vi "Lookup Class by ID (String).vi"(8 "error in (no error)":errorcluster, 11 "Class ID":string) -> (0 "error out":errorcluster, 2 "Found?":bool, 3 "Class Information":T1)   [LabVIEW 2023]
doc: "<b> </b> <b> </b>\n© 2017 Q Software Innovations, LLC\nwritten by Quentin \"Q\" Alldredge\nproduced in LabVIEW 2015\n\nsupport@qsoftwareinnovations.com\nwww.qsoftwareinnovations.com\n\nAll rights reserved.\n\nRedistribution and use in source and binary forms, with or without modification, are permitted provided that the following conditions are met:\n\n * Redistributions of source code must retain the above copyright notice, this list of conditions and the following disclaimer.\n * Redistributions in binary form must reproduce the above copyright notice, this list of conditions and the following disclaimer in the documentation and/or other materials provided with the distribution.\n * Neither the name of Q Software Innovations, LLC. nor the names of its contributors may be used to endorse or promote products derived from this software without specific prior written permission.\n\nTHIS SOFTWARE IS PROVIDED BY THE COPYRIGHT HOLDERS AND CONTRIBUTORS \"AS IS\" AND ANY EXPRESS OR IMPLIED WARRANTIES, INCLUDING, BUT NOT LIMITED TO, THE IMPLIED WARRANTIES OF MERCHANTABILITY AND FITNESS FOR A PARTICULAR PURPOSE ARE DISCLAIMED. IN NO EVENT SHALL THE COPYRIGHT OWNER OR CONTRIBUTORS BE LIABLE FOR ANY DIRECT, INDIRECT, INCIDENTAL, SPECIAL, EXEMPLARY, OR CONSEQUENTIAL DAMAGES (INCLUDING, BUT NOT LIMITED TO, PROCUREMENT OF SUBSTITUTE GOODS OR SERVICES; LOSS OF USE, DATA, OR PROFITS; OR BUSINESS INTERRUPTION) HOWEVER CAUSED AND ON ANY THEORY OF LIABILITY, WHETHER IN CONTRACT, STRICT LIABILITY, OR TORT (INCLUDING NEGLIGENCE OR OTHERWISE) ARISING IN ANY WAY OUT OF THE USE OF THIS SOFTWARE, EVEN IF ADVISED OF THE POSSIBILITY OF SUCH DAMAGE."
panel:
  out "exe time (ms)":u32
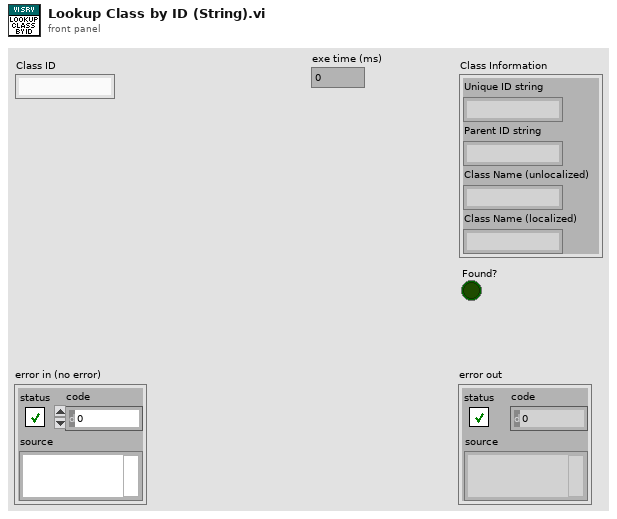
[diagram p1: front panel]
types:
  T1 = cluster{"Unique ID string":string, "Parent ID string":string, "Class Name (unlocalized)":string, "Class Name (localized)":string}
  T2 = cluster{"Unique ID string":string, "Parent ID string":string, "Class Name (unlocalized)":string, "Class Name (localized)":string}[]
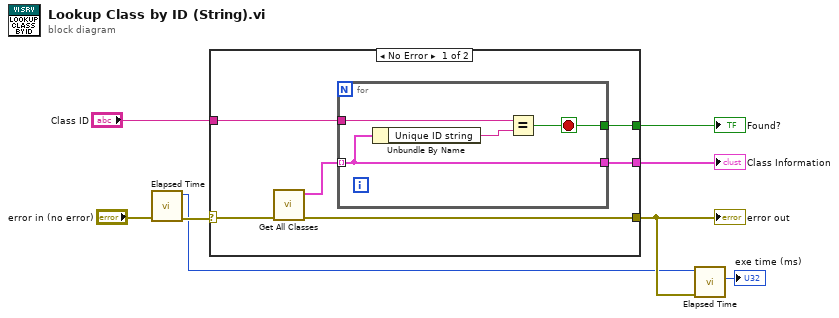
[diagram p0: block diagram]
diagram:
  n1 = call "Elapsed Time.vi"("error in"="error in (no error)") -> ("error out"=w4:errorcluster, "millisecond timer value"=w2:u32)  [unwired: 6 in, 3 out]
  n2 = case shown="No Error" w4 {
    selector: w4 -> [w14 w19]
    tunnel: [w13 w19] -> w3
    tunnel: "Class ID" -> [w11 _]
    tunnel: [w10 _] -> w7
    tunnel: [w9 _] -> w6
    frame No Error {
      n3 = call "Get All Classes.vi"("error in (no error)"=w14) -> ("error out"=w13:errorcluster, "VI Server Classes[]"=w12:T2)  [unwired: 9 in]
      n4 = for {
        tunnel: w12 -> [w18] mode=indexing
        tunnel: w11 -> [w17]
        tunnel: [w18] -> w10
        tunnel: [w15] -> w9
        stop <- w15 stop-if-true
        n5 = Unbundle By Name(w18) -> ("Unique ID string"=w16:string)
        n6 = Equal?(x=w17, y=w16) -> (x = y?=w15:bool)
      }
    }
    frame Error {
    }
  }
  "error out" <- w3
  "Class Information" <- w7
  "Found?" <- w6
  n7 = call "Elapsed Time.vi"("error in"=w3, "past time"=w2) -> ("elapsed time (ms)"=→"exe time (ms)":u32)  [unwired: 5 in, 4 out]
